vi "Modbus Client.vi"() -> ()   [LabVIEW 2015]
doc: "Simple Modbus Client Application."
uses:
  PL Modbus Client.lvclass
panel:
  in  "input registers":T1={"data"=[], "address"=0, "number of items"=8, "read ir"=FALSE} {"number of items" format="%x"; "address" format="%x"; "data" format="%x"}
  in  "single holding register":T2 {"value" format="%x"; "address" format="%x"}
  in  "holding registers":T3={"data"=[], "address"=0, "number of items"=8, "read hr"=FALSE, "write hr"=FALSE} {"number of items" format="%x"; "address" format="%x"; "data" format="%x"}
  in  "discrete inputs":T4={"data"=[], "address"=0, "number of items"=8, "read di"=FALSE} {"number of items" format="%x"; "address" format="%x"}
  in  "single coil":T5 {"address" format="%x"}
  in  "coils":T6={"data"=[], "address"=0, "number of items"=8, "read coils"=FALSE, "write coils"=FALSE} {"number of items" format="%x"; "address" format="%x"}
  in  "timeout, ms":u32=300
  in  "interface":enum32{"serial", "TCP"}(tab)
  in  "serial settings":T7={"port"="", "protocol"=enum."RTU", "address"=1, "baud rate"=9600, "data bits"=8, "parity"=2, "stop bits"=10, "flow control"=0} {"flow control" items=["None", "XON/XOFF", "RTS/CTS", "XON/XOFF & RTS/CTS", "DTR/DSR", "XON/XOFF & DTR/DSR"]; "stop bits" items=["1.0"=10, "1.5"=15, "2.0"=20]; "parity" items=["None", "Odd", "Even", "Mark", "Space"]}
  in  "TCP settings":T8={"ip address"="192.168.1.1", "port"=502, "station address"=255}
  in  "decimal":bool
  in  "stop":bool
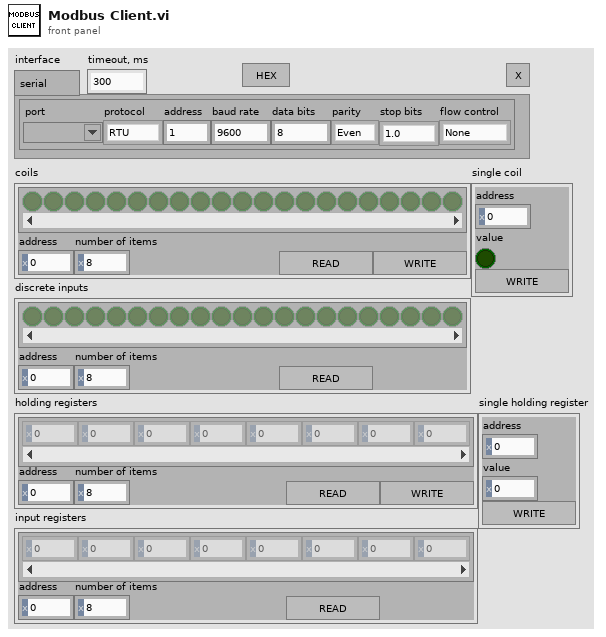
[diagram p1: front panel]
types:
  T1 = cluster{"data":u16[], "address":u16, "number of items":u16, "read ir":bool}
  T2 = cluster{"address":u16, "value":u16, "write single hr":bool}
  T3 = cluster{"data":u16[], "address":u16, "number of items":u16, "read hr":bool, "write hr":bool}
  T4 = cluster{"data":bool[], "address":u16, "number of items":u16, "read di":bool}
  T5 = cluster{"address":u16, "value":bool, "write single coil":bool}
  T6 = cluster{"data":bool[], "address":u16, "number of items":u16, "read coils":bool, "write coils":bool}
  T7 = cluster{"port":refnum<visa-resource-name>, "protocol":enum16{"RTU", "ASCII"}, "address":u8, "baud rate":u32, "data bits":u16, "parity":u16, "stop bits":u16, "flow control":u16}
  T8 = cluster{"ip address":string, "port":u16, "station address":u8}
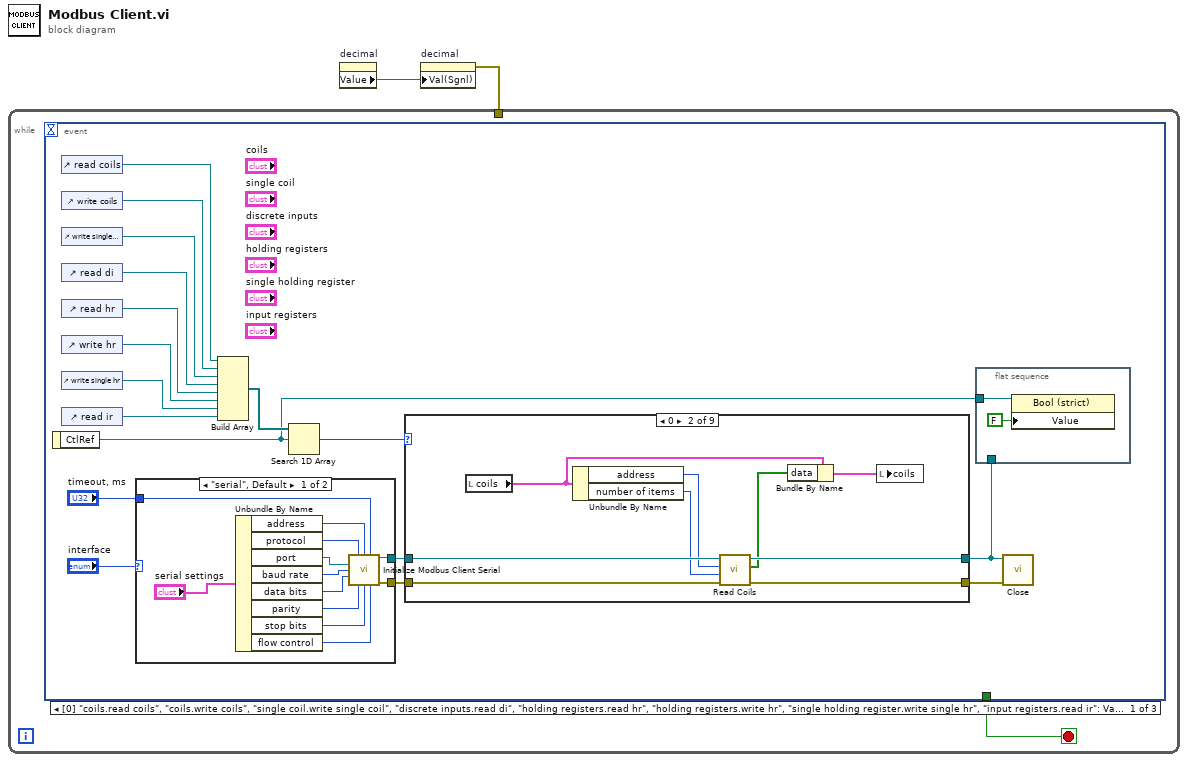
[diagram p0: block diagram]
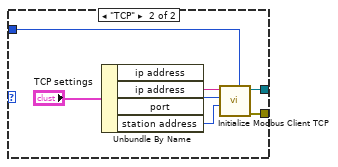
[diagram p2: hidden frame]
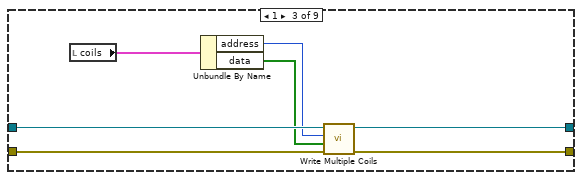
[diagram p4: hidden frame]
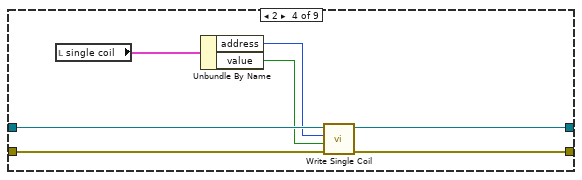
[diagram p5: hidden frame]
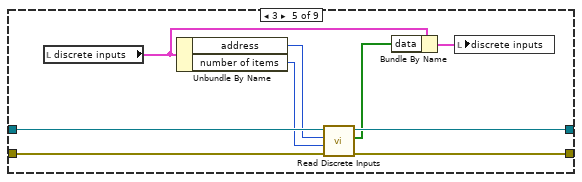
[diagram p6: hidden frame]
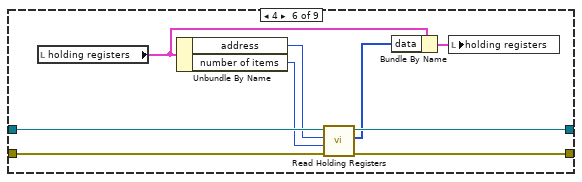
[diagram p7: hidden frame]
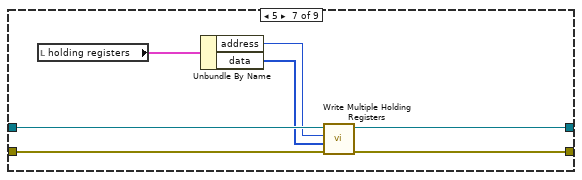
[diagram p8: hidden frame]
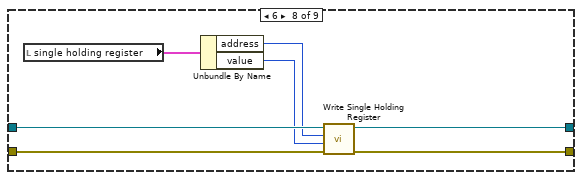
[diagram p9: hidden frame]
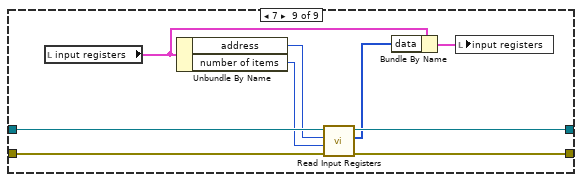
[diagram p10: hidden frame]
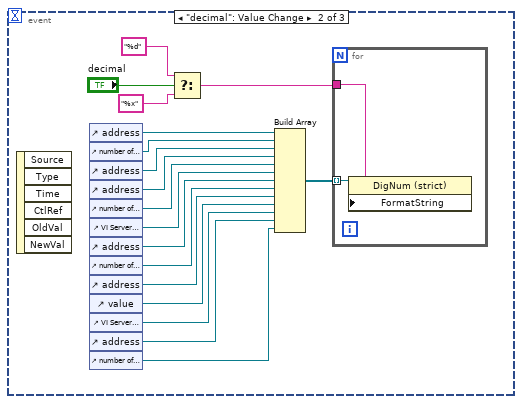
[diagram p11: hidden frame]
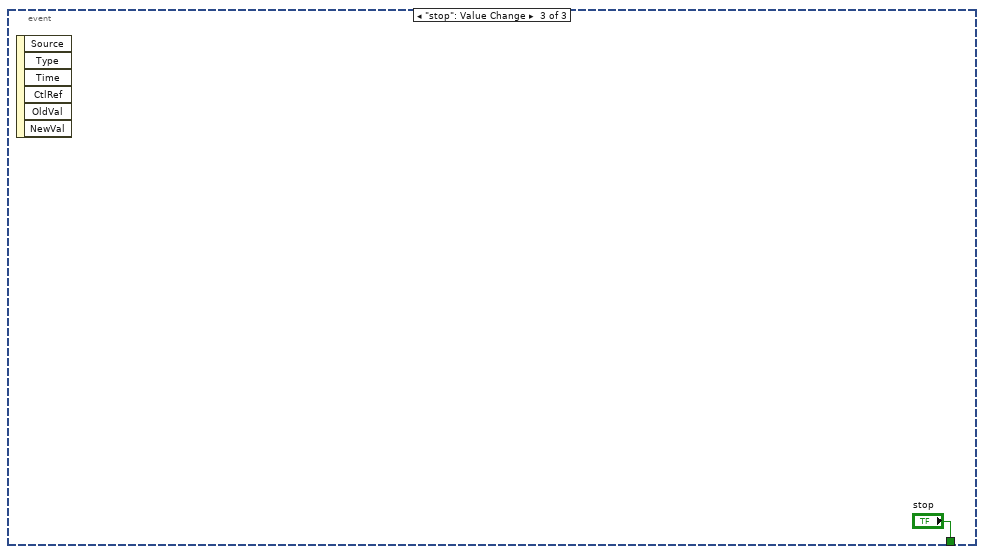
[diagram p12: hidden frame]
diagram:
  n1 = property on="decimal" class="Bool (strict)"() -> ("Value"=w2:bool)  [unwired: 2 in, 2 out]
  n2 = property on="decimal" class="Bool (strict)"("Val(Sgnl)"=w2) -> (error out=w1:errorcluster)  [unwired: 2 in, 1 out]
  n3 = while {
    tunnel: w1 -> [_]
    stop <- w3 stop-if-true
    n4 = event shown="[0] \"coils.read coils\", \"coils.write coils\", \"single coil.write single coil\", \"discrete inputs.read di\", \"holding registers.read hr\", \"holding registers.write hr\", \"single holding register.write single hr\", \"input registers.read ir\": Value Change" {
      selector: _ -> [_ _ _]
      dyn-events: _ -> [_ _ _]
      timeout: _ -> [_ _ _]
      tunnel: [_ _ "stop"] -> w3
      event "coils.read coils", "coils.write coils", "single coil.write single coil", "discrete inputs.read di", "holding registers.read hr", "holding registers.write hr", "single holding register.write single hr", "input registers.read ir": Value Change {
        n5 = event-data() -> ("CtlRef"=w5:refnum<vi>)  [unwired: 1 in]
        n6 = control-ref of="read coils"() -> (w10:refnum<vi>)
        n7 = control-ref of="write coils"() -> (w11:refnum<vi>)
        n8 = control-ref of="write single coil"() -> (w12:refnum<vi>)
        n9 = control-ref of="read di"() -> (w13:refnum<vi>)
        n10 = control-ref of="read hr"() -> (w14:refnum<vi>)
        n11 = control-ref of="write hr"() -> (w15:refnum<vi>)
        n12 = control-ref of="write single hr"() -> (w16:refnum<vi>)
        n13 = control-ref of="read ir"() -> (w17:refnum<vi>)
        n14 = case shown="\"serial\", Default" "interface" {
          tunnel: [w33 w38] -> w6
          tunnel: [w32 w37] -> w7
          tunnel: "timeout, ms" -> [w24 w36]
          frame "serial", Default {
            n15 = Unbundle By Name("serial settings") -> ("address"=w23:u8, "protocol"=w25:enum16{"RTU", "ASCII"}, "port"=w27:refnum<visa-resource-name>, "baud rate"=w26:u32, "data bits"=w28:u16, "parity"=w29:u16, "stop bits"=w30:u16, "flow control"=w31:u16)
            n16 = call "Initialize Modbus Client Serial.vi"("protocol (RTU)"=w25, "station address (1)"=w23, "timeout, ms (300)"=w24, "port"=w27, "baud rate (9600)"=w26, "data bits (8)"=w28, "parity (even)"=w29, "stop bits (1.0)"=w30, "flow control (none)"=w31) -> ("MODBUS out"=w33:refnum<class "PL Modbus Client.lvclass">, "error out"=w32:errorcluster)  [unwired: 5 in]
          }
          frame "TCP" {
            n17 = Unbundle By Name("TCP settings") -> ("ip address"=w40:string, "port"=w39:u16, "station address"=w35:u8)  [unwired: 1 out]
            n18 = call "Initialize Modbus Client TCP.vi"("timeout, ms (300)"=w36, "station address (255)"=w35, "port (502)"=w39, "ip address"=w40) -> ("error out"=w37:errorcluster, "MODBUS out"=w38:refnum<class "PL Modbus Client.lvclass">)  [unwired: 6 in]
          }
        }
        n19 = Build Array(w10, w11, w12, w13, w14, w15, w16, w17) -> (w20:refnum<vi>[])
        n20 = Search 1D Array(1D array=w20, element=w5) -> (index of element=w19:i32)  [unwired: 1 in]
        n21 = case shown="0" w19 {
          tunnel: w6 -> [w43 w52 w59 w66 w75 w84 w91 w98 w107]
          tunnel: [w43 w51 w58 w65 w74 w83 w90 w97 w106] -> w4
          tunnel: w7 -> [w42 w49 w56 w63 w72 w81 w88 w95 w104]
          tunnel: [w42 w50 w57 w64 w73 w82 w89 w96 w105] -> w18
          frame -1, Default {
          }
          frame 0 {
            n22 = local read "coils"() -> (w44:T6)
            n23 = Unbundle By Name(w44) -> ("address"=w47:u16, "number of items"=w46:u16)
            n24 = call "Read Coils.vi"("error in (no error)"=w49, "number of coils"=w46, "address"=w47, "MODBUS in"=w52) -> ("error out"=w50:errorcluster, "values"=w45:bool[], "MODBUS out"=w51:refnum<class "PL Modbus Client.lvclass">)  [unwired: 5 in]
            n25 = Bundle By Name(cluster=w44, "data"=w45) -> (w48:T6)
            n26 = local write "coils"(w48) -> ()
          }
          frame 1 {
            n27 = local read "coils"() -> (w54:T6)
            n28 = Unbundle By Name(w54) -> ("address"=w55:u16, "data"=w53:bool[])
            n29 = call "Write Multiple Coils.vi"("error in (no error)"=w56, "values"=w53, "address"=w55, "MODBUS in"=w59) -> ("error out"=w57:errorcluster, "MODBUS out"=w58:refnum<class "PL Modbus Client.lvclass">)  [unwired: 6 in]
          }
          frame 2 {
            n30 = local read "single coil"() -> (w61:T5)
            n31 = Unbundle By Name(w61) -> ("address"=w62:u16, "value"=w60:bool)
            n32 = call "Write Single Coil.vi"("error in (no error)"=w63, "value"=w60, "address"=w62, "MODBUS in"=w66) -> ("error out"=w64:errorcluster, "MODBUS out"=w65:refnum<class "PL Modbus Client.lvclass">)  [unwired: 6 in]
          }
          frame 3 {
            n33 = local read "discrete inputs"() -> (w67:T4)
            n34 = Unbundle By Name(w67) -> ("address"=w70:u16, "number of items"=w69:u16)
            n35 = call "Read Discrete Inputs.vi"("error in (no error)"=w72, "number of discrete inputs"=w69, "address"=w70, "MODBUS in"=w75) -> ("error out"=w73:errorcluster, "values"=w68:bool[], "MODBUS out"=w74:refnum<class "PL Modbus Client.lvclass">)  [unwired: 5 in]
            n36 = Bundle By Name(cluster=w67, "data"=w68) -> (w71:T4)
            n37 = local write "discrete inputs"(w71) -> ()
          }
          frame 4 {
            n38 = local read "holding registers"() -> (w76:T3)
            n39 = Unbundle By Name(w76) -> ("address"=w79:u16, "number of items"=w78:u16)
            n40 = call "Read Holding Registers.vi"("error in (no error)"=w81, "number of holding registers"=w78, "address"=w79, "MODBUS in"=w84) -> ("error out"=w82:errorcluster, "values"=w77:u16[], "MODBUS out"=w83:refnum<class "PL Modbus Client.lvclass">)  [unwired: 5 in]
            n41 = Bundle By Name(cluster=w76, "data"=w77) -> (w80:T3)
            n42 = local write "holding registers"(w80) -> ()
          }
          frame 5 {
            n43 = local read "holding registers"() -> (w86:T3)
            n44 = Unbundle By Name(w86) -> ("address"=w87:u16, "data"=w85:u16[])
            n45 = call "Write Multiple Holding Registers.vi"("error in (no error)"=w88, "values"=w85, "address"=w87, "MODBUS in"=w91) -> ("error out"=w89:errorcluster, "MODBUS out"=w90:refnum<class "PL Modbus Client.lvclass">)  [unwired: 6 in]
          }
          frame 6 {
            n46 = local read "single holding register"() -> (w93:T2)
            n47 = Unbundle By Name(w93) -> ("address"=w94:u16, "value"=w92:u16)
            n48 = call "Write Single Holding Register.vi"("error in (no error)"=w95, "value"=w92, "address"=w94, "MODBUS in"=w98) -> ("error out"=w96:errorcluster, "MODBUS out"=w97:refnum<class "PL Modbus Client.lvclass">)  [unwired: 6 in]
          }
          frame 7 {
            n49 = local read "input registers"() -> (w99:T1)
            n50 = Unbundle By Name(w99) -> ("address"=w102:u16, "number of items"=w101:u16)
            n51 = call "Read Input Registers.vi"("error in (no error)"=w104, "number of input registers"=w101, "address"=w102, "MODBUS in"=w107) -> ("error out"=w105:errorcluster, "values"=w100:u16[], "MODBUS out"=w106:refnum<class "PL Modbus Client.lvclass">)  [unwired: 5 in]
            n52 = Bundle By Name(cluster=w99, "data"=w100) -> (w103:T1)
            n53 = local write "input registers"(w103) -> ()
          }
        }
        n54 = flat-sequence {
          tunnel: w5 -> [w22]
          tunnel: w4 -> [_]
          frame #0 {
            n55 = property class="Bool (strict)"(reference=w22, "Value"=FALSE) -> ()  [unwired: 1 in, 2 out]
          }
        }
        n56 = call-dynamic "Close.vi"("error in (no error)"=w18, "MODBUS in"=w4) -> ()  [unwired: 9 in, 1 out]
      }
      event "decimal": Value Change {
        n57 = event-data() -> ()  [unwired: 1 in, 6 out]
        n58 = control-ref of="address"() -> (w120:refnum<vi>)
        n59 = control-ref of="number of items"() -> (w119:refnum<vi>)
        n60 = control-ref of="address"() -> (w118:refnum<vi>)
        n61 = control-ref of="address"() -> (w117:refnum<vi>)
        n62 = control-ref of="number of items"() -> (w116:refnum<vi>)
        n63 = control-ref of="VI Server Reference"() -> (w115:refnum<vi>)
        n64 = control-ref of="address"() -> (w114:refnum<vi>)
        n65 = control-ref of="number of items"() -> (w113:refnum<vi>)
        n66 = control-ref of="address"() -> (w112:refnum<vi>)
        n67 = control-ref of="value"() -> (w111:refnum<vi>)
        n68 = control-ref of="VI Server Reference"() -> (w110:refnum<vi>)
        n69 = control-ref of="address"() -> (w109:refnum<vi>)
        n70 = control-ref of="number of items"() -> (w108:refnum<vi>)
        n71 = Select(t="%d", s="decimal", f="%x") -> (s? t:f=w121:string)
        n72 = Build Array(w120, w119, w118, w117, w116, w115, w114, w113, w112, w111, w110, w109, w108) -> (w125:refnum<vi>[])
        n73 = for {
          tunnel: w125 -> [w127] mode=indexing
          tunnel: w121 -> [w126]
          n74 = property class="DigNum (strict)"(reference=w127, "FormatString"=w126) -> ()  [unwired: 1 in, 2 out]
        }
      }
      event "stop": Value Change {
        n75 = event-data() -> ()  [unwired: 1 in, 6 out]
      }
    }
  }
